vi "Main with Notifier.vi"() -> ()   [LabVIEW 2019]
doc: "This template is for the Queued Message Handler design pattern.\n\nThe Event Handling Loop generates messages based on user interface actions.\n\nThe Message Handling Loop processes messages generated by the Event Handling Loop, or by other messages. The messages are string values, so new messages can be added easily to the Message Cases case structure in the Message Handling Loop. Each message cluster can also provide an optional value for Message Data, which is a variant that can be converted to whatever message-specific data is required."
uses:
  <vilib>/ErrorRing/Error Ring.xnode
  controls/UI Data.ctl
  support/Message Queue/Message Queue.lvlib
  <vilib>/Utility/error.llb/Error Cluster From Error Code.vi
  support/User Event - Stop/User Event - Stop.lvlib
  controls/Daqtypedef.ctl
  controls/Acquire Cluster.ctl
  <vilib>/DAQmx/read.llb/DAQmx Read (Analog Wfm 1Chan NSamp).vi
  <vilib>/measure/NI_MAPro.lvlib
  <vilib>/measure/maspectr.llb/FFT Spectrum (Mag-Phase) for 1 Chan.vi
  <vilib>/Analysis/4window.llb/windowTd.ctl
  <vilib>/Analysis/NI_AALPro.lvlib
panel:
  in  "DB ON OFF":bool
  in  "window":T1=1 items=["Rectangle"=0, "Hanning"=1, "Hamming"=2, "Blackman-Harris"=3, "Exact Blackman"=4, "Blackman"=5, "Flat Top"=6, "4 Term B-Harris "=7, "7 Term B-Harris"=8, "Low Sidelobe"=9, "Blackman Nuttall"=11, "Triangle"=30, "Bartlett-Hanning"=31, "Bohman"=32, "Parzen"=33, "Welch"=34, "Kaiser"=60, "Dolph-Chebyshev"=61, "Gaussian"=62]
  in  "Acquisition Configuration":T2
  in  "Stop Acquisition":bool
  in  "Start Acquisition":bool
  in  "Exit":bool
  out "Raw Signal":waveform(dbl)(graph)
  out "Amplitude Spectrum":cluster{"f0":dbl, "df":dbl, "phase":dbl[]}(graph)
  out "Status Line":string
  # "Laboratorium OSP"
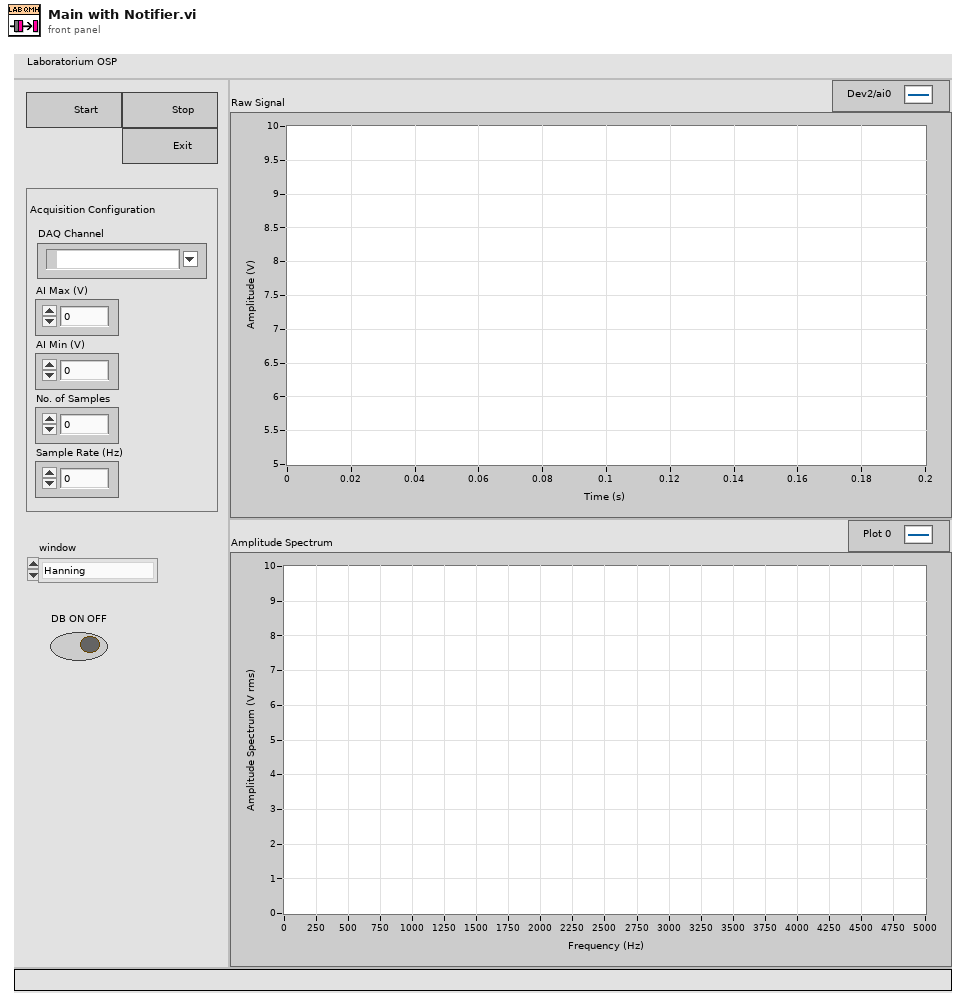
[diagram p1: front panel]
types:
  T1 = typedef "NI_AALPro.lvlib/windowTd.ctl" = u32
  T2 = typedef "Daqtypedef.ctl" = cluster{"PhysicalChanName":tag, "AI.Max":dbl, "AI.Min":dbl, "SampQuant.SampPerChan":i32, "SampClk.Rate":dbl}
  T3 = typedef "Acquire Cluster.ctl" = cluster{"DAQmxChannel":T2, "configData.ini Path":path, "DAQmx Task":refnum<k21>, "TDMS file Path":path}
  T4 = typedef "UI Data.ctl" = cluster{"Start Acquisition":refnum<vi>, "Stop Acquisition":refnum<vi>, "Status Line":refnum<vi>, "Exit":refnum<vi>, "Acquisition Conf":refnum<vi>, "Status Line Message":string}
  T5 = typedef "Message Queue.lvlib/All Message Queues.ctl" = cluster{"UI":refnum<queue>, "Acquire":refnum<queue>}
  T6 = cluster{"dB On (F)":bool, "unwrap phase (F)":bool, "convert to degree (F)":bool}
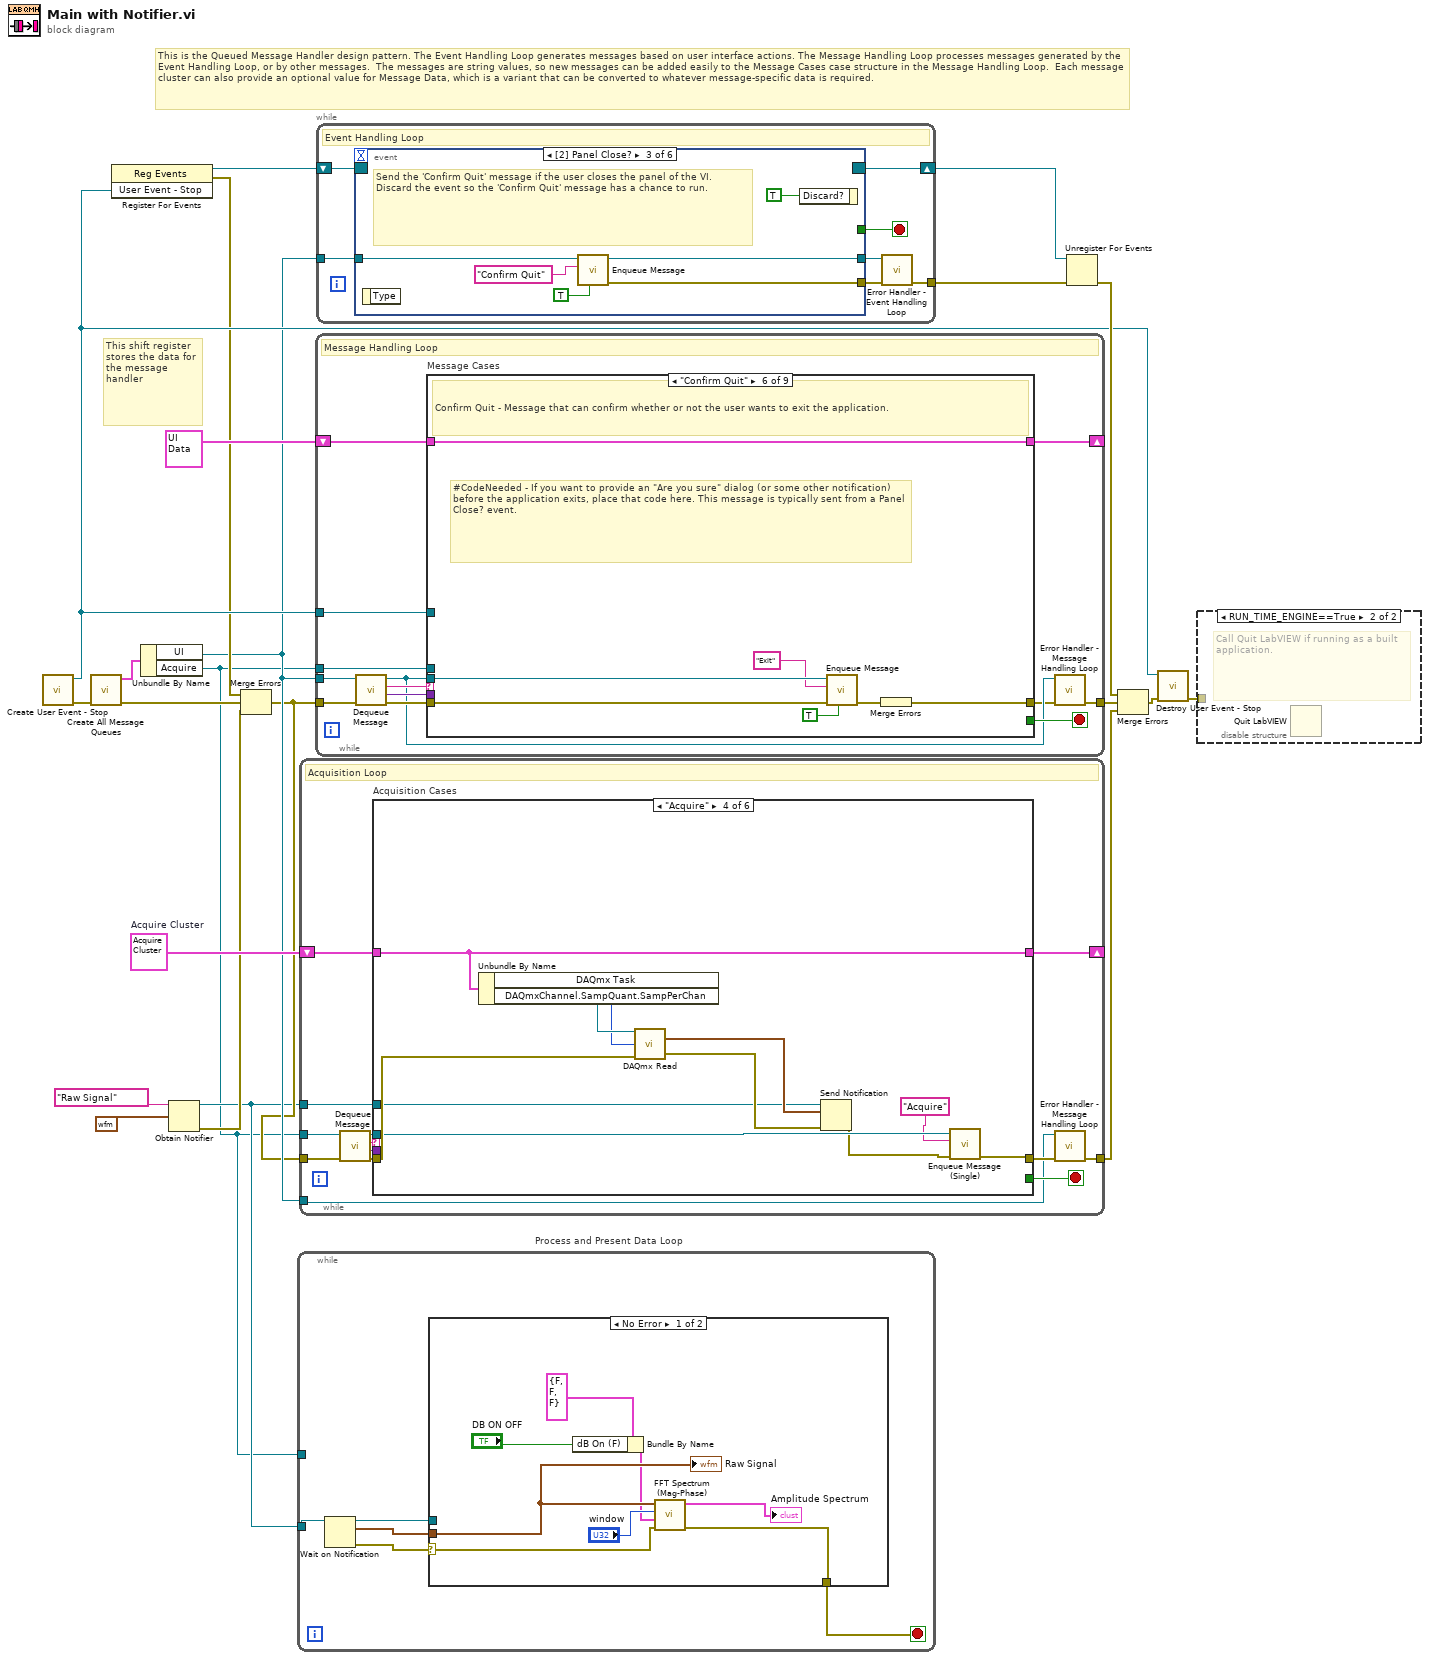
[diagram p0: block diagram]
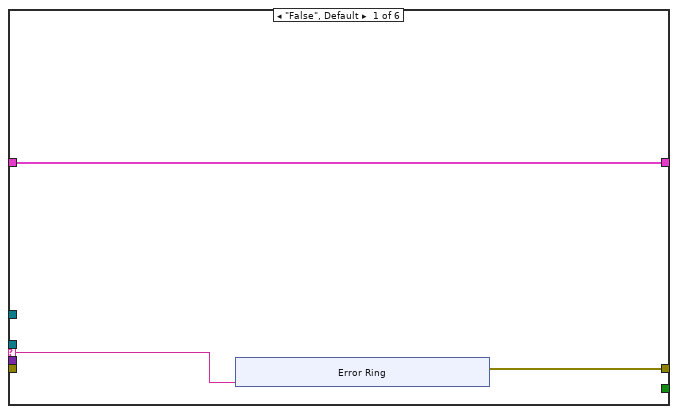
[diagram p3: hidden frame]
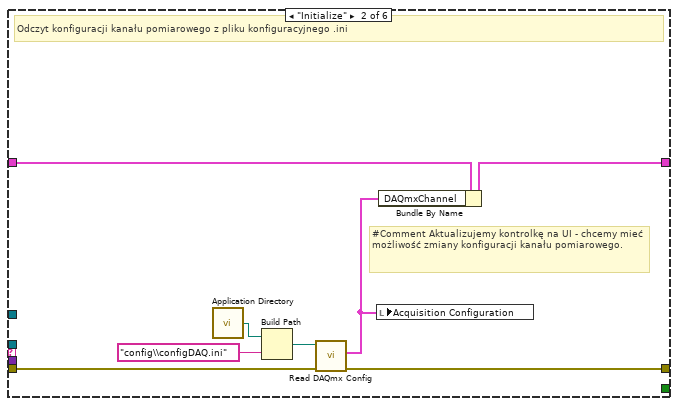
[diagram p4: hidden frame]
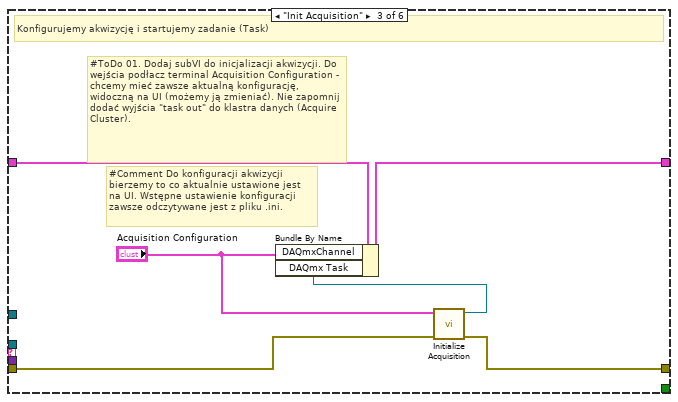
[diagram p5: hidden frame]
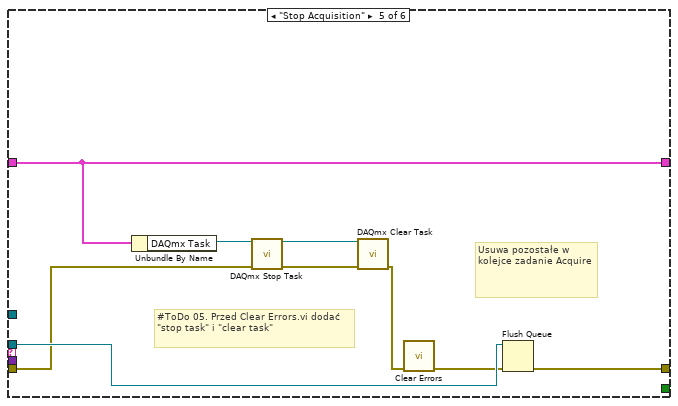
[diagram p6: hidden frame]
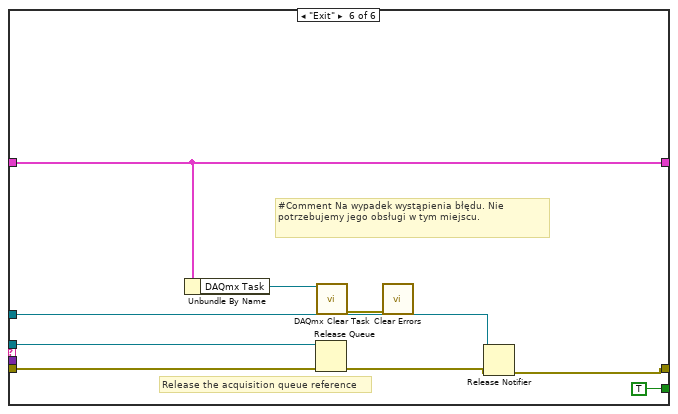
[diagram p7: hidden frame]
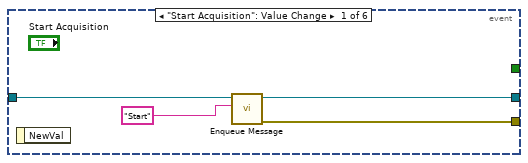
[diagram p9: hidden frame]
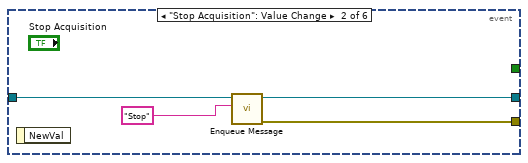
[diagram p10: hidden frame]
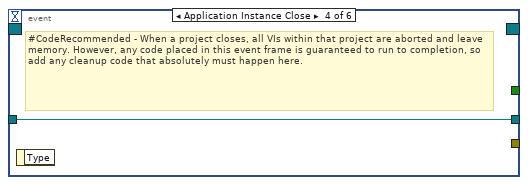
[diagram p11: hidden frame]
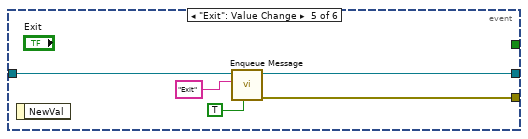
[diagram p12: hidden frame]
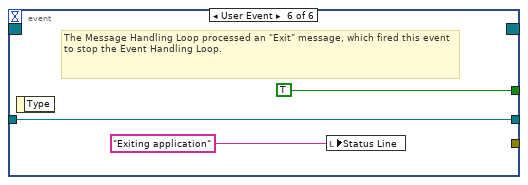
[diagram p13: hidden frame]
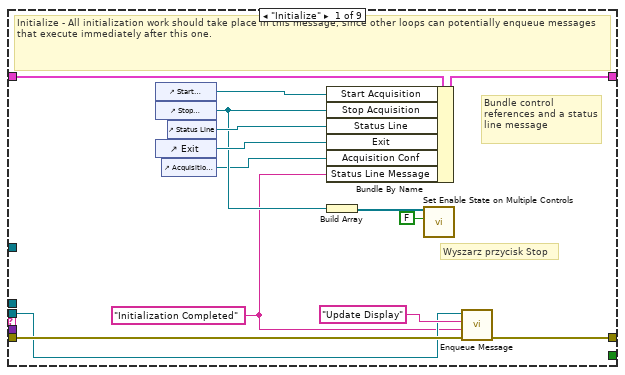
[diagram p14: hidden frame]
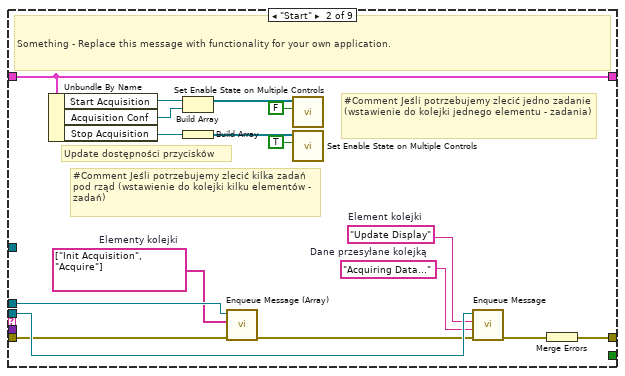
[diagram p15: hidden frame]
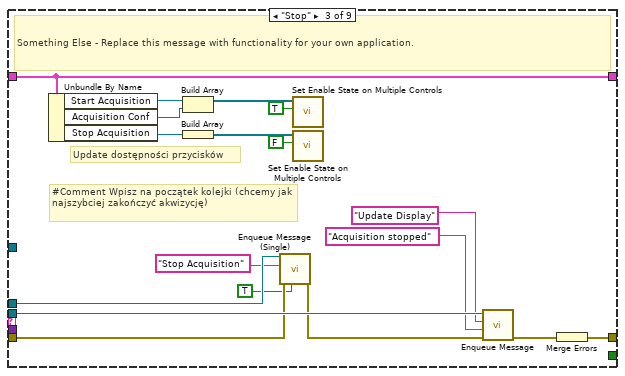
[diagram p16: hidden frame]
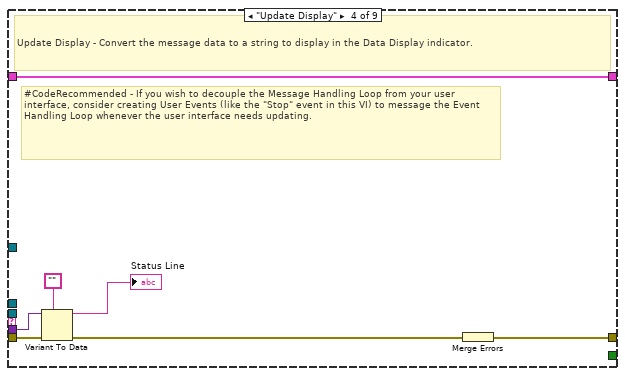
[diagram p17: hidden frame]
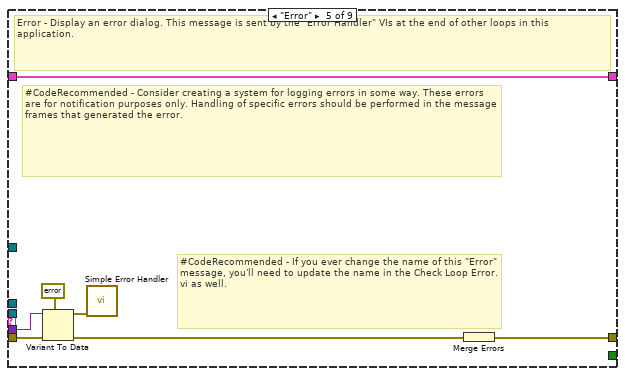
[diagram p18: hidden frame]
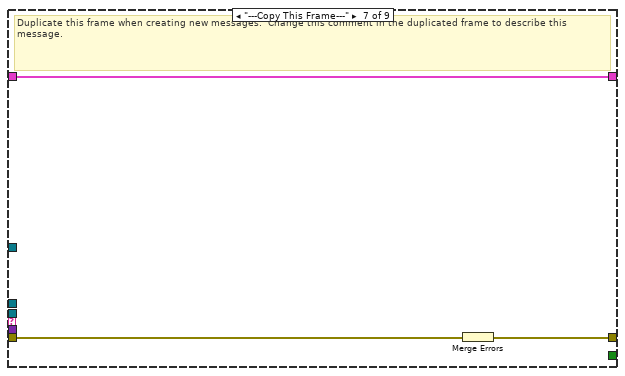
[diagram p19: hidden frame]
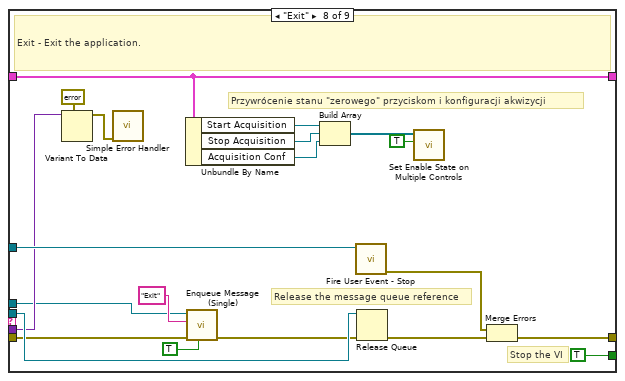
[diagram p20: hidden frame]
diagram:
  w8 = T3 {"DAQmxChannel"={"PhysicalChanName"="", "AI.Max"=0.0, "AI.Min"=0.0, "SampQuant.SampPerChan"=0, "SampClk.Rate"=0.0}, "configData.ini Path"=path "", "DAQmx Task"="", "TDMS file Path"=path ""}  # Acquire Cluster
  # "This is the Queued Message Handler design pattern. The Event Handling Loop generates messages based on user interface actions. The Message Handling Loop processes messages generated by the Event Handling Loop, or by other messages.  The messages are string values, so new messages can be added easily to the Message Cases case structure in the Message Handling Loop.  Each message cluster can also provide an optional value for Message Data, which is a variant that can be converted to whatever message-specific data is required."
  # "This shift register stores the data for the message handler"
  n1 = call "Create User Event - Stop.vi"() -> ("error out"=w19:errorcluster, "User Event - Stop"=w11:refnum<user-event>)  [unwired: 10 in]
  n2 = call "Create All Message Queues.vi"("error in (no error)"=w19) -> ("error out"=w22:errorcluster, "Message Queues out"=w21:T5)  [unwired: 9 in]
  n3 = register-events(w11) -> (reference out=w12:refnum<event-registration>, error out=w10:errorcluster)  [unwired: 2 in]
  n4 = Unbundle By Name(w21) -> ("UI"=w7:refnum<queue>, "Acquire"=w1:refnum<queue>)
  n5 = Obtain Notifier(name (unnamed)="Raw Signal", notification data type=waveform(dbl) {"t0"=timestamp(0 s since 1904-01-01), "dt"=0.0, "Y"=[]} ("data")) -> (notifier out=w2:refnum<notifier>, error out=w3:errorcluster)  [unwired: 2 in, 1 out]
  n6 = Merge Errors(w10, w22, w3) -> (w5:errorcluster)
  n7 = while "Process and Present Data Loop" {
    tunnel: w2 -> [w27]
    tunnel: w1 -> [_]
    stop <- w23 stop-if-true
    n8 = Wait on Notification(notifier=w27) -> (notifier out=w26:refnum<notifier>, notification=w25:waveform(dbl), error out=w24:errorcluster)  [unwired: 3 in, 1 out]
    n9 = case shown="No Error" w24 {
      selector: w24 -> [w35 w36]
      tunnel: w26 -> [_ _]
      tunnel: w25 -> [w33 _]
      tunnel: [w32 w36] -> w23
      frame No Error {
        n10 = Bundle By Name(cluster=T6 {"dB On (F)"=FALSE, "unwrap phase (F)"=FALSE, "convert to degree (F)"=FALSE} ("view"), "dB On (F)"="DB ON OFF") -> (w28:T6)
        n11 = call-poly <vilib>:"FFT Spectrum (Mag-Phase).vi"("error in (no error)"=w35, "view"=w28, "window"="window", "time signal"=w33) -> ("error out"=w32:errorcluster, "magnitude"=→"Amplitude Spectrum":cluster{"f0":dbl, "df":dbl, "magnitude":dbl[]})  [unwired: 3 in, 3 out]
        "Raw Signal" <- w33
      }
      frame Error {
      }
    }
  }
  n12 = while {
    tunnel: w5 -> [w48]
    tunnel: w1 -> [w47]
    tunnel: [w43] -> w9
    shift-right: [w40] -> _
    shift-left: w8 -> [w41]
    tunnel: w7 -> [w38]
    tunnel: w2 -> [w37]
    stop <- w42 stop-if-true
    # "Acquisition Loop"
    n13 = call "Dequeue Message.vi"("error in (no error)"=w48, "Message Queue"=w47) -> ("error out"=w46:errorcluster, "Message Data"=w45:variant, "Message"=w49:string, "dup Message Queue"=w39:refnum<queue>)  [unwired: 6 in]
    n14 = case "Acquisition Cases" shown="\"Acquire\"" w49 {
      selector: w49 -> [w52 _ _ _ _ _]
      tunnel: w46 -> [_ w67 w72 w83 w85 w101]
      tunnel: w45 -> [_ _ _ _ _ _]
      tunnel: w39 -> [_ _ _ w79 w93 w100]
      tunnel: [w51 w66 w73 w80 w87 w95] -> w44
      tunnel: [_ _ _ _ _ TRUE] -> w42
      tunnel: w41 -> [w50 w62 w70 w84 w91 w98]
      tunnel: [w50 w60 w71 w84 w91 w98] -> w40
      tunnel: w37 -> [_ _ _ w74 _ w94]
      frame "False", Default {
        n15 = xnode "Error Ring"("parameter 0"=w52) -> ("error out"=w51:errorcluster)
      }
      frame "Initialize" {
        # "#Comment Aktualizujemy kontrolkę na UI - chcemy mieć możliwość zmiany konfiguracji kanału pomiarowego."
        # "Odczyt konfiguracji kanału pomiarowego z pliku konfiguracyjnego .ini"
        n16 = call <vilib>:"Application Directory.vi"() -> ("Application Directory"=w65:path)
        n17 = Build Path(base path=w65, name or relative path="config\\configDAQ.ini") -> (appended path=w63:path)
        n18 = call "Read DAQmx Config.vi"("error in (no error)"=w67, "configuration file path"=w63) -> ("error out"=w66:errorcluster, "DAQmx Channel out"=w61:T2)  [unwired: 7 in, 1 out]
        n19 = local write "Acquisition Configuration"(w61) -> ()
        n20 = Bundle By Name(cluster=w62, "DAQmxChannel"=w61) -> (w60:T3)
      }
      frame "Init Acquisition" {
        # "#ToDo 01. Dodaj subVI do inicjalizacji akwizycji. Do wejścia podłacz terminal Acquisition Configuration - chcemy mieć zawsze aktualną konfigurację, widoczną na UI (możemy ją zmieniać). Nie zapomnij dodać wyjścia \"task out\" do klastra danych (Acquire Cluster)."
        # "#Comment Do konfiguracji akwizycji bierzemy to co aktualnie ustawione jest na UI. Wstępne ustawienie konfiguracji zawsze odczytywane jest z pliku .ini."
        # "Konfigurujemy akwizycję i startujemy zadanie (Task)"
        n21 = call "Initialize Acquisition.vi"("error in"=w72, "DAQmxChannel"="Acquisition Configuration") -> ("error out"=w73:errorcluster, "task out"=w68:refnum<k21>)  [unwired: 8 in]
        n22 = Bundle By Name(cluster=w70, "DAQmxChannel"="Acquisition Configuration", "DAQmx Task"=w68) -> (w71:T3)
      }
      frame "Acquire" {
        n23 = Unbundle By Name(w84) -> ("DAQmx Task"=w82:refnum<k21>, "DAQmxChannel.SampQuant.SampPerChan"=w81:i32)
        n24 = call-poly <vilib>:"DAQmx Read.vi"("task/channels in"=w82, "number of samples per channel"=w81, "error in"=w83) -> ("data"=w77:waveform(dbl), "error out"=w76:errorcluster)  [unwired: 10 in, 1 out]
        n25 = Send Notification(notification=w77, notifier=w74, error in (no error)=w76) -> (error out=w75:errorcluster)  [unwired: 1 out]
        n26 = call "Enqueue Message (Single).vi"("error in (no error)"=w75, "Message"="Acquire", "Message Queue"=w79) -> ("error out"=w80:errorcluster)  [unwired: 7 in, 1 out]
      }
      frame "Stop Acquisition" {
        # "#ToDo 05. Przed Clear Errors.vi dodać \"stop task\" i \"clear task\""
        # "Usuwa pozostałe w kolejce zadanie Acquire"
        n27 = Unbundle By Name(w91) -> ("DAQmx Task"=w90:refnum<k21>)
        n28 = call <vilib>:"DAQmx Stop Task.vi"("task/channels in"=w90, "error in"=w85) -> ("task out"=w89:refnum<k21>, "error out"=w88:errorcluster)  [unwired: 12 in]
        n29 = call <vilib>:"DAQmx Clear Task.vi"("task in"=w89, "error in"=w88) -> ("error out"=w86:errorcluster)  [unwired: 13 in]
        n30 = call <vilib>:"Clear Errors.vi"("error in (no error)"=w86) -> ("error out"=w92:errorcluster)  [unwired: 5 in, 1 out]
        n31 = Flush Queue(queue=w93, error in (no error)=w92) -> (error out=w87:errorcluster)  [unwired: 2 out]
      }
      frame "Exit" {
        # "#Comment Na wypadek wystąpienia błędu. Nie potrzebujemy jego obsługi w tym miejscu."
        # "Release the acquisition queue reference"
        n32 = Unbundle By Name(w98) -> ("DAQmx Task"=w97:refnum<k21>)
        n33 = Release Queue(queue=w100, error in (no error)=w101) -> (error out=w96:errorcluster)  [unwired: 1 in, 2 out]
        n34 = call <vilib>:"DAQmx Clear Task.vi"("task in"=w97) -> ("error out"=w99:errorcluster)  [unwired: 14 in]
        n35 = call <vilib>:"Clear Errors.vi"("error in (no error)"=w99) -> ()  [unwired: 5 in, 2 out]
        n36 = Release Notifier(notifier=w94, error in (no error)=w96) -> (error out=w95:errorcluster)  [unwired: 1 in, 2 out]
      }
    }
    n37 = call "Error Handler - Message Handling Loop.vi"("error in (no error)"=w44, "Message Queue"=w38) -> ("dup error in"=w43:errorcluster)  [unwired: 8 in, 1 out]
  }
  n38 = while {
    tunnel: w7 -> [w107]
    shift-right: [w114] -> _
    shift-left: T4 {"Start Acquisition"=refnum, "Stop Acquisition"=refnum, "Status Line"=refnum, "Exit"=refnum, "Acquisition Conf"=refnum, "Status Line Message"=""} ("Data Cluster") -> [w115]
    tunnel: w11 -> [w112]
    tunnel: w5 -> [w111]
    tunnel: [w105] -> w20
    tunnel: w1 -> [w103]
    stop <- w113 stop-if-true
    # "Message Handling Loop"
    n39 = call "Dequeue Message.vi"("error in (no error)"=w111, "Message Queue"=w107) -> ("error out"=w110:errorcluster, "Message Data"=w108:variant, "Message"=w109:string, "dup Message Queue"=w106:refnum<queue>)  [unwired: 6 in]
    n40 = case "Message Cases" shown="\"Confirm Quit\"" w109 {
      selector: w109 -> [_ _ _ _ _ _ _ _ w209]
      tunnel: w106 -> [w121 w144 w162 _ _ w181 _ w208 _]
      tunnel: w110 -> [w128 w140 w158 w169 w178 w185 w188 w198 _]
      tunnel: [w129 w146 w164 w170 w172 w183 w186 w205 w210] -> w104
      tunnel: w115 -> [w127 w137 w148 w171 w177 w184 w187 w193 w211]
      tunnel: [w126 w137 w148 w171 w177 w184 w187 w193 w211] -> w114
      tunnel: [_ _ _ _ _ _ _ TRUE _] -> w113
      tunnel: w108 -> [_ _ _ w168 w176 _ _ w200 _]
      tunnel: w112 -> [_ _ _ _ _ _ _ w204 _]
      tunnel: w103 -> [_ w139 w157 _ _ _ _ w196 _]
      frame "Initialize" {
        w117 = "Initialization Completed" ("Initial Message")
        # "Wyszarz przycisk Stop"
        # "Bundle control references and a status line message"
        # "Initialize - All initialization work should take place in this message, since other loops can potentially enqueue messages that execute immediately after this one."
        n41 = control-ref of="Start Acquisition"() -> (w125:refnum<vi>)
        n42 = control-ref of="Stop Acquisition"() -> (w119:refnum<vi>)
        n43 = control-ref of="Exit"() -> (w123:refnum<vi>)
        n44 = control-ref of="Acquisition Configuration"() -> (w116:refnum<vi>)
        n45 = control-ref of="Status Line"() -> (w124:refnum<vi>)
        n46 = Bundle By Name(cluster=w127, "Start Acquisition"=w125, "Stop Acquisition"=w119, "Status Line"=w124, "Exit"=w123, "Acquisition Conf"=w116, "Status Line Message"=w117) -> (w126:T4)
        n47 = Build Array(w119) -> (w118:refnum<vi>[])
        n48 = call "Set Enable State on Multiple Controls.vi"("Enable?"=FALSE, "Controls"=w118) -> ()  [unwired: 10 in]
        n49 = call-poly "Enqueue Message.vi"("error in (no error)"=w128, "Message Data"=w117, "Message"="Update Display", "Message Queue"=w121) -> ("error out"=w129:errorcluster)  [unwired: 6 in, 1 out]
      }
      frame "Start" {
        w138 = string[] ["Init Acquisition", "Acquire"]  # Elementy kolejki
        w143 = "Update Display"  # Element kolejki
        w142 = "Acquiring Data..."  # Dane przesyłane kolejką
        # "Update dostępności przycisków"
        # "#Comment Jeśli potrzebujemy zlecić jedno zadanie (wstawienie do kolejki jednego elementu - zadania)"
        # "#Comment Jeśli potrzebujemy zlecić kilka zadań pod rząd (wstawienie do kolejki kilku elementów - zadań)"
        # "Something - Replace this message with functionality for your own application."
        n50 = Unbundle By Name(w137) -> ("Start Acquisition"=w136:refnum<vi>, "Acquisition Conf"=w130:refnum<vi>, "Stop Acquisition"=w135:refnum<vi>)
        n51 = Build Array(w136, w130) -> (w134:refnum<vi>[])
        n52 = Build Array(w135) -> (w133:refnum<vi>[])
        n53 = call "Enqueue Message (Array).vi"("error in (no error)"=w140, "Message Array"=w138, "Message Queue"=w139) -> ("error out"=w141:errorcluster)  [unwired: 7 in, 1 out]
        n54 = call "Set Enable State on Multiple Controls.vi"("Enable?"=FALSE, "Controls"=w134) -> ()  [unwired: 10 in]
        n55 = call "Set Enable State on Multiple Controls.vi"("Enable?"=TRUE, "Controls"=w133) -> ()  [unwired: 10 in]
        n56 = call-poly "Enqueue Message.vi"("error in (no error)"=w141, "Message Data"=w142, "Message"=w143, "Message Queue"=w144) -> ("error out"=w145:errorcluster)  [unwired: 6 in, 1 out]
        n57 = Merge Errors(w145) -> (w146:errorcluster)
      }
      frame "Stop" {
        # "Update dostępności przycisków"
        # "#Comment Wpisz na początek kolejki (chcemy jak najszybciej zakończyć akwizycję)"
        # "Something Else - Replace this message with functionality for your own application."
        n58 = Unbundle By Name(w148) -> ("Start Acquisition"=w154:refnum<vi>, "Acquisition Conf"=w147:refnum<vi>, "Stop Acquisition"=w153:refnum<vi>)
        n59 = Build Array(w154, w147) -> (w152:refnum<vi>[])
        n60 = Build Array(w153) -> (w151:refnum<vi>[])
        n61 = call "Enqueue Message (Single).vi"("Priority Message? (F)"=TRUE, "error in (no error)"=w158, "Message"="Stop Acquisition", "Message Queue"=w157) -> ("error out"=w159:errorcluster)  [unwired: 6 in, 1 out]
        n62 = call "Set Enable State on Multiple Controls.vi"("Enable?"=TRUE, "Controls"=w152) -> ()  [unwired: 10 in]
        n63 = call "Set Enable State on Multiple Controls.vi"("Enable?"=FALSE, "Controls"=w151) -> ()  [unwired: 10 in]
        n64 = call-poly "Enqueue Message.vi"("error in (no error)"=w159, "Message Data"="Acquisition stopped" ("\"Do Something Else\" button pressed"), "Message"="Update Display", "Message Queue"=w162) -> ("error out"=w163:errorcluster)  [unwired: 6 in, 1 out]
        n65 = Merge Errors(w163) -> (w164:errorcluster)
      }
      frame "Update Display" {
        # "#CodeRecommended - If you wish to decouple the Message Handling Loop from your user interface, consider creating User Events (like the \"Stop\" event in this VI) to message the Event Handling Loop whenever the user interface needs updating."
        # "Update Display - Convert the message data to a string to display in the Data Display indicator."
        n66 = Variant To Data(error in=w169, type="", Variant=w168) -> (data=→"Status Line":string, error out=w166:errorcluster)
        n67 = Merge Errors(w166) -> (w170:errorcluster)
      }
      frame "Error" {
        # "#CodeRecommended - If you ever change the name of this \"Error\" message, you'll need to update the name in the Check Loop Error.vi as well."
        # "#CodeRecommended - Consider creating a system for logging errors in some way. These errors are for notification purposes only. Handling of specific errors should be performed in the message frames that generated the error."
        # "Error - Display an error dialog. This message is sent by the \"Error Handler\" VIs at the end of other loops in this application."
        n68 = Variant To Data(error in=w178, type=errorcluster {"status"=FALSE, "code"=0, "source"=""} ("error constant"), Variant=w176) -> (data=w174:errorcluster, error out=w173:errorcluster)
        n69 = call <vilib>:"Simple Error Handler.vi"("error in (no error)"=w174) -> ()  [unwired: 4 in, 5 out]
        n70 = Merge Errors(w173) -> (w172:errorcluster)
      }
      frame "Confirm Quit" {
        # "#CodeNeeded - If you want to provide an \"Are you sure\" dialog (or some other notification) before the application exits, place that code here. This message is typically sent from a Panel Close? event."
        # "Confirm Quit - Message that can confirm whether or not the user wants to exit the application."
        n71 = call-poly "Enqueue Message.vi"("Priority Message? (F)"=TRUE, "error in (no error)"=w185, "Message"="Exit", "Message Queue"=w181) -> ("error out"=w182:errorcluster)  [unwired: 6 in, 1 out]
        n72 = Merge Errors(w182) -> (w183:errorcluster)
      }
      frame "---Copy This Frame---" {
        # "Duplicate this frame when creating new messages.  Change this comment in the duplicated frame to describe this message."
        n73 = Merge Errors(w188) -> (w186:errorcluster)
      }
      frame "Exit" {
        # "Przywrócenie stanu \"zerowego\" przyciskom i konfiguracji akwizycji"
        # "Stop the VI"
        # "Release the message queue reference"
        # "Exit - Exit the application."
        n74 = Variant To Data(type=errorcluster {"status"=FALSE, "code"=0, "source"=""} ("error constant"), Variant=w200) -> (data=w201:errorcluster)  [unwired: 1 in, 1 out]
        n75 = call <vilib>:"Simple Error Handler.vi"("error in (no error)"=w201) -> ()  [unwired: 4 in, 5 out]
        n76 = Unbundle By Name(w193) -> ("Start Acquisition"=w192:refnum<vi>, "Stop Acquisition"=w191:refnum<vi>, "Acquisition Conf"=w189:refnum<vi>)
        n77 = call "Enqueue Message (Single).vi"("Priority Message? (F)"=TRUE, "error in (no error)"=w198, "Message"="Exit", "Message Queue"=w196) -> ("error out"=w199:errorcluster)  [unwired: 6 in, 1 out]
        n78 = Build Array(w192, w191, w189) -> (w194:refnum<vi>[])
        n79 = call "Fire User Event - Stop.vi"("User Event - Stop"=w204) -> ("error out"=w203:errorcluster)  [unwired: 10 in]
        n80 = Release Queue(queue=w208, error in (no error)=w199) -> (error out=w206:errorcluster)  [unwired: 1 in, 2 out]
        n81 = call "Set Enable State on Multiple Controls.vi"("Enable?"=TRUE, "Controls"=w194) -> ()  [unwired: 10 in]
        n82 = Merge Errors(w203, w206) -> (w205:errorcluster)
      }
      frame Default {
        # "'Default' case only runs if there is a message that isn't defined in any of the other cases.  Output a programming error."
        n83 = xnode "Error Ring"("parameter 0"=w209) -> ("error out"=w210:errorcluster)
      }
    }
    n84 = call "Error Handler - Message Handling Loop.vi"("error in (no error)"=w104, "Message Queue"=w106) -> ("dup error in"=w105:errorcluster)  [unwired: 8 in, 1 out]
  }
  n85 = while {
    tunnel: w7 -> [w225]
    shift-right: [w223] -> w16
    shift-left: w12 -> [w224]
    tunnel: [w219] -> w13
    stop <- w221 stop-if-true
    # "Event Handling Loop"
    n86 = event shown="[2] Panel Close?" {
      selector: w224 -> [_ _ _ _ _ _]
      dyn-events: [_ _ _ _ _ _] -> w223
      timeout: _ -> [_ _ _ _ _ _]
      tunnel: [_ _ _ _ _ TRUE ("Discard?")] -> w221
      tunnel: w225 -> [w229 w233 w238 w240 w245 w248]
      tunnel: [w226 w230 w237 _ w244 _] -> w222
      tunnel: [w228 w232 w236 w240 w243 w248] -> w220
      event "Start Acquisition": Value Change {
        n87 = event-data() -> ()  [unwired: 1 in, 1 out]
        n88 = call-poly "Enqueue Message.vi"("Message"="Start", "Message Queue"=w229) -> ("error out"=w226:errorcluster, "dup Message Queue"=w228:refnum<queue>)  [unwired: 8 in]
      }
      event "Stop Acquisition": Value Change {
        n89 = event-data() -> ()  [unwired: 1 in, 1 out]
        n90 = call-poly "Enqueue Message.vi"("Message"="Stop", "Message Queue"=w233) -> ("error out"=w230:errorcluster, "dup Message Queue"=w232:refnum<queue>)  [unwired: 8 in]
      }
      event Panel Close? {
        # "Send the 'Confirm Quit' message if the user closes the panel of the VI. Discard the event so the 'Confirm Quit' message has a chance to run."
        n91 = event-data() -> ()  [unwired: 1 in, 1 out]
        n92 = call-poly "Enqueue Message.vi"("Priority Message? (F)"=TRUE, "Message"="Confirm Quit", "Message Queue"=w238) -> ("error out"=w237:errorcluster, "dup Message Queue"=w236:refnum<queue>)  [unwired: 7 in]
        n93 = event-data("Discard?"=TRUE) -> ()  [unwired: 1 in, 1 out]
      }
      event Application Instance Close {
        # "#CodeRecommended - When a project closes, all VIs within that project are aborted and leave memory. However, any code placed in this event frame is guaranteed to run to completion, so add any cleanup code that absolutely must happen here."
        n94 = event-data() -> ()  [unwired: 1 in, 1 out]
      }
      event "Exit": Value Change {
        n95 = event-data() -> ()  [unwired: 1 in, 1 out]
        n96 = call-poly "Enqueue Message.vi"("Priority Message? (F)"=TRUE, "Message"="Exit", "Message Queue"=w245) -> ("error out"=w244:errorcluster, "dup Message Queue"=w243:refnum<queue>)  [unwired: 7 in]
      }
      event User Event {
        # "The Message Handling Loop processed an \"Exit\" message, which fired this event to stop the Event Handling Loop."
        n97 = event-data() -> ()  [unwired: 1 in, 1 out]
        n98 = local write "Status Line"("Exiting application" ("VI Stopped")) -> ()
      }
    }
    n99 = call "Error Handler - Event Handling Loop.vi"("error in (no error)"=w222, "Message Queue"=w220) -> ("dup error in"=w219:errorcluster)  [unwired: 8 in, 1 out]
  }
  n100 = Unregister For Events(event registration refnum=w16, error in=w13) -> (error out=w17:errorcluster)
  n101 = Merge Errors(w17, w20, w9) -> (w18:errorcluster)
  n102 = call "Destroy User Event - Stop.vi"("error in (no error)"=w18, "User Event - Stop"=w11) -> ("error out"=w14:errorcluster)  [unwired: 9 in]
  n103 = disable-structure shown="RUN_TIME_ENGINE==True" {
    disable-tunnel: w14 -> [_ _]
    frame condition #0 (active) {
    }
    frame condition #1 {
      # "Call Quit LabVIEW if running as a built application."
      n104 = Quit LabVIEW() -> ()  [unwired: 1 in]
    }
  }
